vi "TCP read to CRLF.vi"(8 "error in":errorcluster, 9 "timeout":i32, 10 "bytes to read":i32, 11 "connection ID":refnum<k5>) -> (0 "error out":errorcluster, 1 "timed out?":bool, 2 "data":u8[](array[numeric]))   [LabVIEW 2021, in "TCP Shared Components.lvlib"]
doc: "This function reads a TCP string from the bus up until a CRLF and checks for errors. It is a wrapper for standard functionality."
uses:
  TCP Shared Components.lvlib
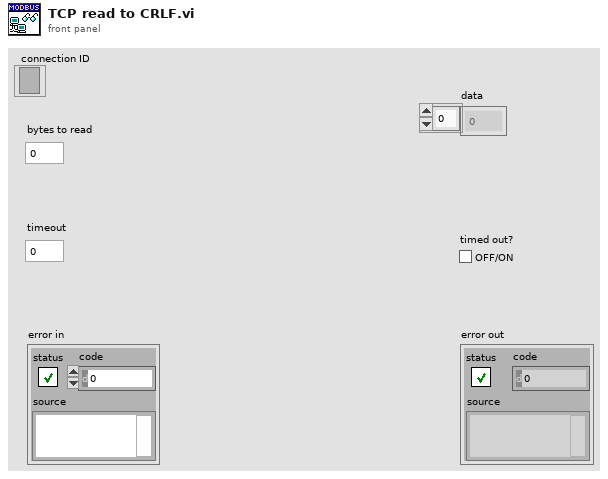
[diagram p1: front panel]
types:
  T1 = enum16{"Standard", "Buffered", "CRLF", "Immediate"}
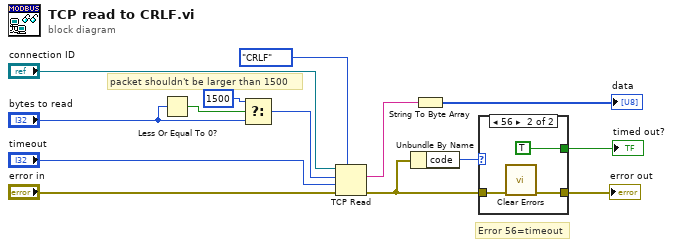
[diagram p0: block diagram]
diagram:
  # "packet shouldn't be larger than 1500"
  # "Error 56=timeout"
  n1 = Less Or Equal To 0?(x="bytes to read") -> (x <= 0?=w3:bool)
  n2 = Select(t=1500, s=w3, f="bytes to read") -> (s? t:f=w6:i32)
  n3 = TCP Read(connection ID="connection ID", bytes to read=w6, error in (no error)="error in", 7:T1."CRLF" ("mode (standard)"), 9:"timeout") -> (data out=w1:string, error out=w7:errorcluster)  [unwired: 1 out]
  n4 = Unbundle By Name(w7) -> ("code"=w2:i32)
  n5 = String To Byte Array(string=w1) -> (unsigned byte array=→"data":u8[])
  n6 = case shown="56" w2 {
    tunnel: w7 -> [w15 w18]
    tunnel: [w15 w17] -> w14
    tunnel: [_ TRUE] -> w10
    frame 0, Default {
    }
    frame 56 {
      n7 = call <vilib>:"Clear Errors.vi"("error in (no error)"=w18) -> ("error out"=w17:errorcluster)  [unwired: 5 in, 1 out]
    }
  }
  "error out" <- w14
  "timed out?" <- w10
